vi "Stop Core.vi"(10 "final error code":i32, 11 "DAQmx Actor in":refnum<class "DAQmx Actor.lvclass">) -> (3 "DAQmx Actor out":refnum<class "DAQmx Actor.lvclass">)   [LabVIEW 2024, in "DAQmx Actor.lvlib" / "DAQmx Actor.lvclass"]
doc: "<p>(<strong>Filename</strong>: <span class=\"dnl\">Actor Framework.lvlib:Actor.lvclass:Stop Core.vi</span>)</p>\n<p>Defines what the actor does before it stops. Use the <strong>final error code</strong> input to determine whether the actor shut down in response to an error.</p>\n<p>By default, this method passes the Stop message along to all <a href=\"nihelplauncher://docs/csh?context=lvcore_lvcomm_af_launch_nested_actor\">auto-stop nested actors</a>. A descendant class may override this method to define additional behavior, such as shutting down any processes the actor initiated in its override of the <a href=\"nihelplauncher://docs/csh?context=lvcore_lvcomm_af_actor_core\">Actor Core</a> method.</p>"
uses:
  DAQmx Actor.lvclass
  <vilib>/ActorFramework/Actor/Actor.lvclass
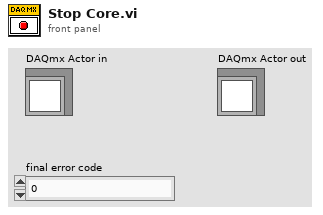
[diagram p1: front panel]
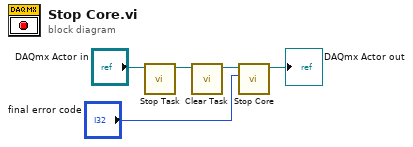
[diagram p0: block diagram]
diagram:
  n1 = call "Stop Task.vi"("DAQmx Actor in"="DAQmx Actor in") -> ("DAQmx Actor out"=w2:refnum<class "DAQmx Actor.lvclass">)  [unwired: 9 in, 1 out]
  n2 = call "Clear Task.vi"("DAQmx Actor in"=w2) -> ("DAQmx Actor out"=w1:refnum<class "DAQmx Actor.lvclass">)  [unwired: 9 in, 1 out]
  n3 = call-parent "Stop Core.vi"("final error code"="final error code", "Actor in"=w1) -> ("Actor out"=→"DAQmx Actor out":refnum<class "DAQmx Actor.lvclass">)  [unwired: 9 in]
